vi "Get Paragraphs.Text.vi"(8 "error in (no error)":errorcluster, 11 "xwpfDocument in":refnum<class "xwpfDocument.lvclass">) -> (0 "error out":errorcluster, 2 "Paragraphs.Text":string[](array[string]), 3 "xwpfDocument out":refnum<class "xwpfDocument.lvclass">)   [LabVIEW 2017, in "Word_Specific.lvlib" / "xwpfDocument.lvclass"]
uses:
  xwpfDocument.lvclass
  xwpfDocument.lvclass/xwpfDocument.ctl
  xwpfParagraph/Get Runs.Text.vi
  xwpfParagraph/xwpfParagraph.lvclass
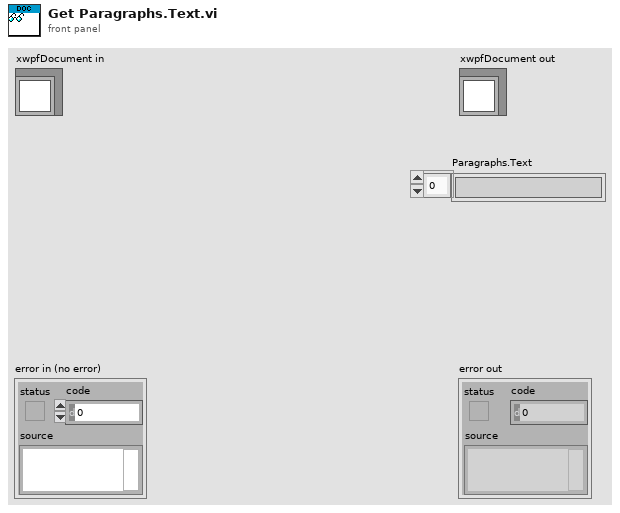
[diagram p1: front panel]
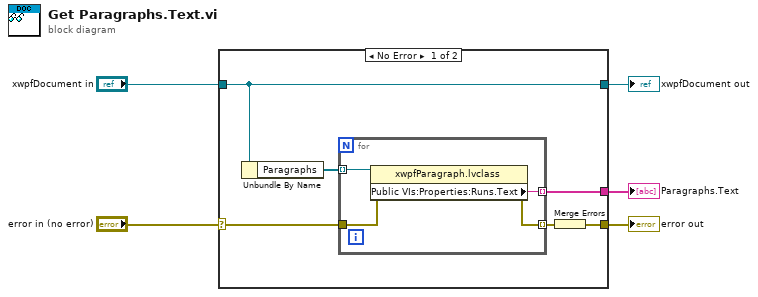
[diagram p0: block diagram]
diagram:
  n1 = case shown="No Error" "error in (no error)" {
    selector: "error in (no error)" -> [w6 w16]
    tunnel: [w7 w16] -> w4
    tunnel: [w11 w17] -> w2
    tunnel: "xwpfDocument in" -> [w11 w17]
    tunnel: [w9 _] -> w1
    frame No Error {
      n2 = Unbundle By Name(w11) -> ("Paragraphs"=w10:refnum<class "xwpfParagraph.lvclass">[])
      n3 = for {
        tunnel: w10 -> [w15] mode=indexing
        tunnel: [w14] -> w9 mode=indexing
        tunnel: [w13] -> w8 mode=indexing
        tunnel: w6 -> [w12]
        n4 = property class="xwpfParagraph.lvclass"(reference=w15, error in=w12) -> (error out=w13:errorcluster, "Public VIs:Properties:Runs.Text"=w14:string)  [unwired: 1 out]
      }
      n5 = Merge Errors(w8) -> (w7:errorcluster)
    }
    frame Error {
    }
  }
  "error out" <- w4
  "xwpfDocument out" <- w2
  "Paragraphs.Text" <- w1
